vi "tdmsProperties.vi"(4 "AnalogSettings":T1=[{"AnalogOut (Volt)"=[5.0, 5.0, 5.0, 5.0], "DAQmx Device Name"="PXI1Slot2"}, {"AnalogOut (Volt)"=[5.0, 5.0, 5.0, 5.0], "DAQmx Device Name"="PXI1Slot3"}, {"AnalogOut (Volt)"=[5.0, 5.0, 5.0, 5.0], "DAQmx Device Name"="PXI1Slot6"}] caption="Analog Output Voltage Setup", 5 "TDMS Group Name":string, 6 "AnalogInSettings":T2[](array[typedef])=[{"Input Voltage Range"=10.0, "Upsample Coefficient"=1, "Analog Input Channels"="PXI1Slot2/ai0:7", "Configuration"=10106}, {"Input Voltage Range"=10.0, "Upsample Coefficient"=1, "Analog Input Channels"="PXI1Slot3/ai0:7", "Configuration"=10106}, {"Input Voltage Range"=10.0, "Upsample Coefficient"=2, "Analog Input Channels"="PXI1Slot6/ai0:4", "Configuration"=10106}] caption="Analog Input Tasks per PXI device" {"Configuration" items=["Differential"=10106, "RSE"=10083, "NRSE"=10078, "Pseudodifferential"=12529]}, 7 "HWSettings":T3={"Nr. of Columns"=1, "Nr. of Rows"=18, "OverSampling"=10, "Fetch Rate "=20, "Sampling Rate"=50000, "Nr. of BNC inputs"=3, "Sample Strip Length"=10} caption="Hardware Settingss", 8 "Error In":errorcluster, 10 "LUT":i32[](array[numeric]) caption="Channel Mix Vector", 11 "tdms file In":refnum<k34>) -> (0 "Error Out":errorcluster, 3 "tdms file Out":refnum<k34>)   [LabVIEW 2012]
uses:
  controls/General Hardware config.ctl
  controls/DAQ Setup.ctl
  controls/AnalogOutputSetup.ctl
panel:
  # "Array"
  # "Acq. System"
  # "Other analog Input"
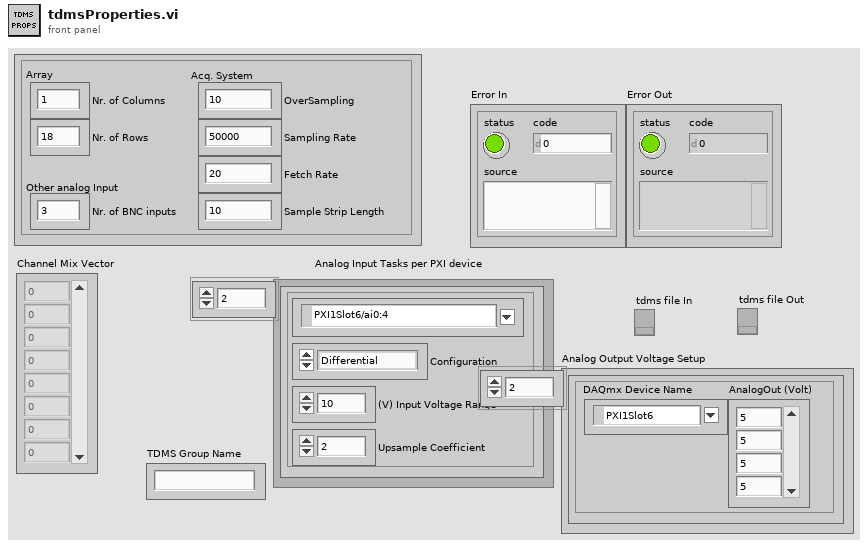
[diagram p1: front panel]
types:
  T1 = typedef "AnalogOutputSetup.ctl" = cluster{"AnalogOut (Volt)":dbl[], "DAQmx Device Name":tag}[]
  T2 = typedef "DAQ Setup.ctl" = cluster{"Input Voltage Range":dbl, "Upsample Coefficient":u32, "Analog Input Channels":tag, "Configuration":i32}
  T3 = typedef "General Hardware config.ctl" = cluster{"Nr. of Columns":i32, "Nr. of Rows":i32, "OverSampling":i32, "Fetch Rate ":i32, "Sampling Rate":i32, "Nr. of BNC inputs":i32, "Sample Strip Length":i32}
  T4 = typedef "LVStringsAndValuesArrayTypeDef_I32.ctl" = cluster{"String":string, "Value":i32}[]
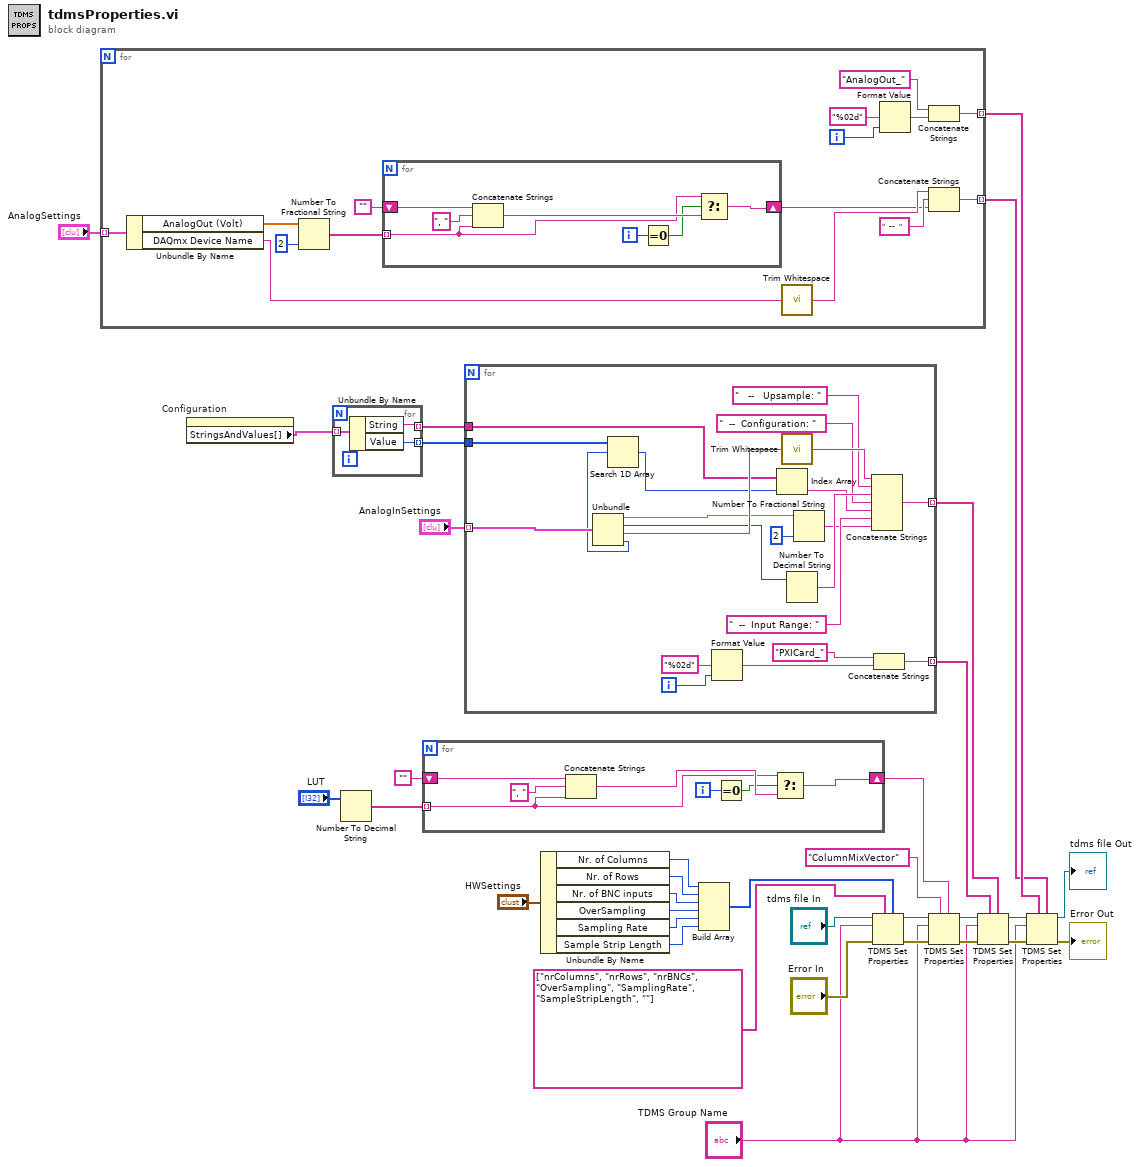
[diagram p0: block diagram]
diagram:
  n1 = for {
    tunnel: "AnalogSettings" -> [w45] mode=indexing
    tunnel: [w36] -> w7 mode=indexing
    tunnel: [w35] -> w8 mode=indexing
    i -> [w48]
    n2 = Unbundle By Name(w45) -> ("AnalogOut (Volt)"=w40:dbl[], "DAQmx Device Name"=w44:tag)
    n3 = Number To Fractional String(number=w40, precision (6)=i16 2) -> (F-format string=w39:string[])  [unwired: 2 in]
    n4 = for {
      tunnel: w39 -> [w50] mode=indexing
      shift-right: [w54] -> w37
      shift-left: "" -> [w56]
      i -> [w52]
      n5 = Concatenate Strings(w56, ", " ("string"), w50) -> (w53:string)
      n6 = Equal To 0?(x=w52) -> (x = 0?=w51:bool)
      n7 = Select(t=w50, s=w51, f=w53) -> (s? t:f=w54:string)
    }
    n8 = call <vilib>:"Trim Whitespace.vi"("string"=w44) -> ("trimmed string"=w43:string)  [unwired: 1 in]
    n9 = Format Value(format string="%02d", value (0)=w48) -> (output string=w47:string)  [unwired: 1 in]
    n10 = Concatenate Strings("AnalogOut_" ("string"), w47) -> (w35:string)
    n11 = Concatenate Strings(w43, "  --  " ("string"), w37) -> (w36:string)
  }
  n12 = property on="Configuration" class="Ring (strict)"() -> ("StringsAndValues[]"=w5:T4)  [unwired: 2 in, 2 out]
  n13 = for {
    tunnel: w5 -> [w59] mode=indexing
    tunnel: [w58] -> w3 mode=indexing
    tunnel: [w57] -> w4 mode=indexing
    n14 = Unbundle By Name(w59) -> ("String"=w57:string, "Value"=w58:i32)
  }
  n15 = Number To Decimal String(number="LUT") -> (decimal integer string=w23:string[])  [unwired: 1 in]
  n16 = for {
    tunnel: w23 -> [w60] mode=indexing
    shift-right: [w64] -> w21
    shift-left: "" -> [w66]
    i -> [w62]
    n17 = Concatenate Strings(w66, ", " ("string"), w60) -> (w63:string)
    n18 = Equal To 0?(x=w62) -> (x = 0?=w61:bool)
    n19 = Select(t=w60, s=w61, f=w63) -> (s? t:f=w64:string)
  }
  n20 = for {
    tunnel: "AnalogInSettings" -> [w83] mode=indexing
    tunnel: [w84] -> w15 mode=indexing
    tunnel: [w77] -> w14 mode=indexing
    tunnel: w4 -> [w68]
    tunnel: w3 -> [w69]
    i -> [w87]
    n21 = Unbundle(w83) -> ("Input Voltage Range"=w73:dbl, "Upsample Coefficient"=w79:u32, "Analog Input Channels"=w82:tag, "Configuration"=w70:i32)
    n22 = Search 1D Array(1D array=w69, element=w70) -> (index of element=w67:i32)  [unwired: 1 in]
    n23 = Format Value(format string="%02d", value (0)=w87) -> (output string=w86:string)  [unwired: 1 in]
    n24 = Index Array(array=w68, index=w67) -> (element=w75:string)
    n25 = call <vilib>:"Trim Whitespace.vi"("string"=w82) -> ("trimmed string"=w81:string)  [unwired: 1 in]
    n26 = Number To Decimal String(number=w79) -> (decimal integer string=w78:string)  [unwired: 1 in]
    n27 = Number To Fractional String(number=w73, precision (6)=i16 2) -> (F-format string=w71:string)  [unwired: 2 in]
    n28 = Concatenate Strings(w81, "   --   Upsample: " ("string"), w78, "  --  Configuration: " ("string"), w75, "  --  Input Range: " ("string"), w71) -> (w77:string)
    n29 = Concatenate Strings("PXICard_", w86) -> (w84:string)
  }
  n30 = Unbundle By Name("HWSettings") -> ("Nr. of Columns"=w32:i32, "Nr. of Rows"=w31:i32, "Nr. of BNC inputs"=w30:i32, "OverSampling"=w29:i32, "Sampling Rate"=w28:i32, "Sample Strip Length"=w27:i32)
  n31 = Build Array(w32, w31, w30, w29, w28, w27) -> (w2:i32[])
  n32 = TDMS Set Properties(5:w2, 7:string[] ["nrColumns", "nrRows", "nrBNCs", "OverSampling", "SamplingRate", "SampleStripLength", ""], 8:"Error In", 10:"TDMS Group Name", 11:"tdms file In") -> (0:w24:errorcluster, 3:w19:refnum<k34>)  [unwired: 1 in, 2 out]
  n33 = TDMS Set Properties(5:w21, 7:"ColumnMixVector" ("property names"), 8:w24, 10:"TDMS Group Name", 11:w19) -> (0:w17:errorcluster, 3:w16:refnum<k34>)  [unwired: 1 in, 2 out]
  n34 = TDMS Set Properties(5:w14, 7:w15, 8:w17, 10:"TDMS Group Name", 11:w16) -> (0:w12:errorcluster, 3:w11:refnum<k34>)  [unwired: 1 in, 2 out]
  n35 = TDMS Set Properties(5:w7, 7:w8, 8:w12, 10:"TDMS Group Name", 11:w11) -> (0:→"Error Out":errorcluster, 3:→"tdms file Out":refnum<k34>)  [unwired: 1 in, 2 out]
